vi "G#Object_UserCounterState.vi"(0 "reference in":refnum<class "G#Object.lvclass">, 2 "user counter (F)":bool, 5 "error in (no error)":errorcluster) -> (14 "reference out":refnum<class "G#Object.lvclass">, 19 "error out":errorcluster)   [LabVIEW 2020, in "G#Object.lvclass"]
doc: "Set the state of the user counter for the object. If disabled, the next Destroy execution of the object will kill the object."
uses:
  G#Object.lvclass
  G#Object.lvclass/G#Object.ctl
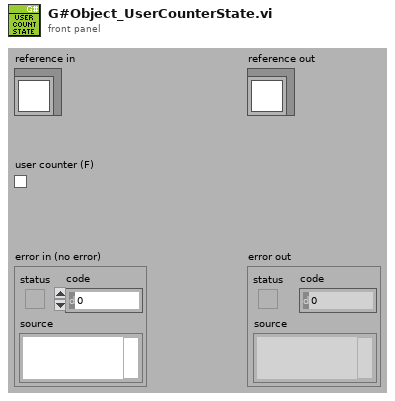
[diagram p1: front panel]
types:
  T1 = typedef "G#Object.lvclass/G#Object_ObjectInfoType.ctl" = cluster{"ObjectName":string, "ObjectID":u32, "Users":i32, "Counter":bool, "AttributeRefs":u32[], "FullClassName":string, "ClassName":string, "CreateMethod":T2, "GenericDestructorExists":bool, "Owner":string}
  T2 = typedef "G#Object.lvclass/G#Object_CreateMethod.ctl" = enum16{"Create", "Create or look up existing", "Look up existing"}
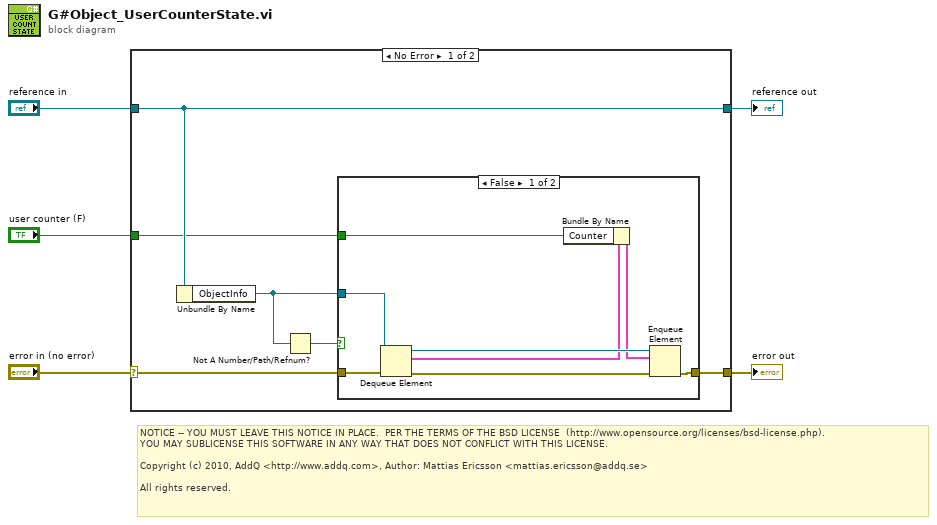
[diagram p0: block diagram]
diagram:
  # "NOTICE -- YOU MUST LEAVE THIS NOTICE IN PLACE.  PER THE TERMS OF THE BSD LICENSE  (http://www.opensource.org/licenses/bsd-license.php).\nYOU MAY SUBLICENSE THIS SOFTWARE IN ANY WAY THAT DOES NOT CONFLICT WITH THIS LICENSE.\n\nCopyright (c) 2010, AddQ <http://www.addq.com>, Author: Mattias Ericsson <mattias.ericsson@addq.se>\n\nAll rights reserved."
  n1 = case shown="No Error" "error in (no error)" {
    selector: "error in (no error)" -> [w11 w22]
    tunnel: [w10 w22] -> w4
    tunnel: [w9 w21] -> w2
    tunnel: "reference in" -> [w9 w21]
    tunnel: "user counter (F)" -> [w6 _]
    frame No Error {
      n2 = Unbundle By Name(w9) -> ("ObjectInfo"=w8:refnum<queue>)
      n3 = Not A Number/Path/Refnum?(number/path/refnum=w8) -> (NaN/Path/Refnum?=w7:bool)
      n4 = case shown="False" w7 {
        tunnel: w11 -> [w19 w20]
        tunnel: [w15 w20] -> w10
        tunnel: w8 -> [w18 _]
        tunnel: w6 -> [w12 _]
        frame False {
          n5 = Dequeue Element(queue=w18, error in (no error)=w19) -> (queue out=w16:refnum<queue>, element=w13:T1, error out=w17:errorcluster)  [unwired: 1 in, 1 out]
          n6 = Bundle By Name(cluster=w13, "Counter"=w12) -> (w14:T1)
          n7 = Enqueue Element(queue=w16, element=w14, error in (no error)=w17) -> (error out=w15:errorcluster)  [unwired: 1 in, 2 out]
        }
        frame True {
        }
      }
    }
    frame Error {
    }
  }
  "error out" <- w4
  "reference out" <- w2
